vi "Untitled 1.vi"   [LabVIEW 2016]
uses:
  Classes/Workspace/Fixture.lvclass
  Classes/Workspace/Component/Component Tray.lvclass
  Classes/Workspace/Carrier Tray/Assembly Tray.lvclass
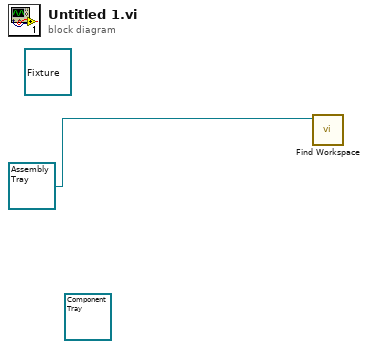
[diagram p0: block diagram]
diagram:
  (unwired) refnum<class "Component Tray.lvclass"> refnum ("Component Tray.lvclass")
  (unwired) refnum<class "Fixture.lvclass"> refnum ("Fixture.lvclass")
  n1 = call-dynamic "Find Workspace.vi"("Carrier Tray in"=refnum<class "Assembly Tray.lvclass"> refnum ("Assembly Tray.lvclass")) -> ()  [unwired: 7 in, 4 out]
